vi "http handle header.vi"(7 "continuation":bool, 9 "header field data":string, 10 "header field name":string, 11 "application request in":T1) -> (3 "application request out":T1)   [LabVIEW 2013, in "Basic HTTP server.lvclass"]
uses:
  Basic HTTP server.lvclass
  http request.ctl
  http method.ctl
  HTTP headers/http header data.ctl
  HTTP headers/http headers.lvlib
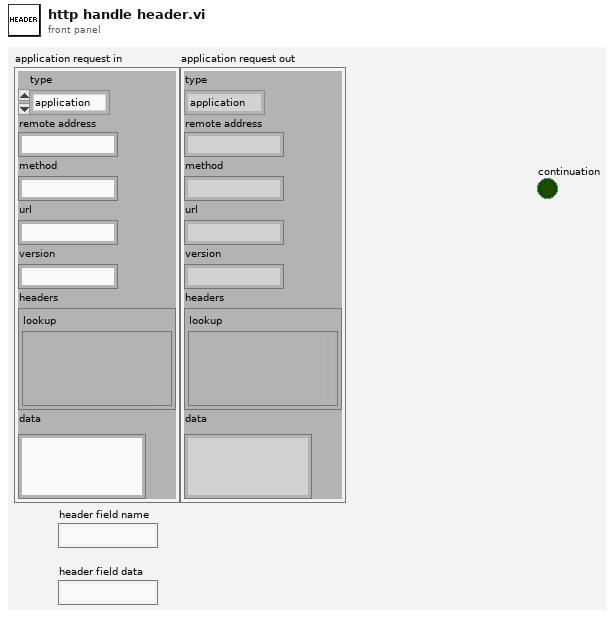
[diagram p1: front panel]
types:
  T1 = typedef "Basic HTTP server.lvclass/http request.ctl" = cluster{"type":T2, "remote address":string, "method":string, "url":string, "version":string, "headers":T3, "data":string}
  T2 = typedef "Basic HTTP server.lvclass/http method.ctl" = enum16{"application", "error", "upgrade", "expect"}
  T3 = typedef "http headers.lvlib/http header data.ctl" = cluster{"lookup":variant}
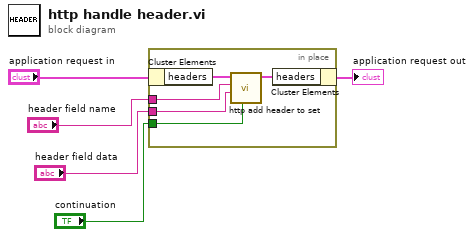
[diagram p0: block diagram]
diagram:
  n1 = in-place {
    in-place-border: "header field data" -> [w10]
    in-place-border: "header field name" -> [w9]
    in-place-border: "continuation" -> [w8]
    n2 = in-place-cluster #1("application request in") -> ("headers"=w7:T3)
    n3 = call "http add header to set.vi"("continuation?"=w8, "header field data"=w10, "header field name"=w9, "headers in"=w7) -> ("headers out"=w6:T3)  [unwired: 7 in]
    n4 = in-place-cluster #1("headers"=w6) -> (→"application request out":T1)
  }
